vi "Shooter_Hood_Homing.vi"(0 "MotorConfig":T2={"CAN Address"=0, "Invert"=FALSE, "InvertSensor"=FALSE, "Unit Conversion Factor"=0.0, "Brake Mode"=enum."Override to Brake", "Reverse Limt Switch Mode"=enum."Disabled", "Forward Limt Swith Mode"=enum."Disabled", "PWM Channel"=enum."Invalid", "Motor Controller Type"=enum."Talon SRX", "Peak Current (A)"=0, "Continuous Current (A)"=0, "Peak Duration (ms)"=0, "Current Limit Enable"=FALSE}, 1 "Hood_Motor_DevRef":T7={"DeviceStatus"={"status"=FALSE, "code"=0, "source"=""}, "Type"=enum."PWM", "PWM"={"PWM Channel"=enum."Invalid", "DeadBand"={"Name"="", "maxPositivePwm"=0, "minPositivePwm"=0, "centerPwm"=0, "maxNegativePwm"=0, "minNegativePwm"=0, "angularRange"=0}}, "CAN"={"Device Number"=0, "SetOutput VI Ref"=variant(enum8{"Percent VBus", "Current", "Speed", "Position", "Voltage"} enum."Percent VBus"), "GetOutput VI Ref"=variant(refnum<k1> refnum), "Enable VI Ref"=variant(dbl 12.0), "Disable VI Ref"=variant(enum8{"Percent VBus", "Speed", "Position", "Slave", "Unchanged / Invalid", "Voltage Compensation", "Current", "Motion Profile"} enum."Percent VBus"), "Data"=variant}, "Invert"=FALSE, "DIO PWM"={"PWM \"Enable\" Channel"=enum."Invalid", "DIOChannel"=enum."Invalid", "PWM Rate"=0.0}}, 2 "Reset":bool, 3 "Homing Activated":bool, 4 "Controller_Command":dbl) -> (5 "Motor_Output":dbl, 6 "Homing_State":T1)   [LabVIEW 2019]
uses:
  <vilib>/Rock Robotics/WPI/MotorControl/WPI_MotorControlDeviceRef.ctl
  <vilib>/Rock Robotics/WPI/MotorControl/WPI_MotorControlType.ctl
  <vilib>/Rock Robotics/SystemInterfaces/DIO/FPGA_DIOPWMChannel.ctl
  <vilib>/Rock Robotics/WPI/PWM/WPI_PWMDeadband.ctl
  <vilib>/Rock Robotics/SystemInterfaces/DIO/FPGA_DIOChannel.ctl
  ArgosLib/Config/ConfigComponents/TypeDefs/Config_Motor.ctl
  <vilib>/Rock Robotics/WPI/ThirdParty/Phoenix-LabVIEW/Motor Controller/Controls/CTRE_Phoenix_MotorControl_NeutralMode.ctl
  <vilib>/Rock Robotics/WPI/ThirdParty/Phoenix-LabVIEW/Motor Controller/Controls/CTRE_Phoenix_MotorControl_LimitSwitchNormal.ctl
  ArgosLib/Config/ConfigComponents/TypeDefs/Config_MotorCtrlType.ctl
  TypeDefs/Hood_Homing_State.ctl
  ArgosLib/Signal Processing/TypeDefs/EdgeDetector_Type.ctl
  <vilib>/Rock Robotics/WPI/ThirdParty/Phoenix-LabVIEW/Motor Controller/Get/CTRE_Phoenix_MotorController_GetSupplyAndStatorCurrent_Enhanced.vi
  <vilib>/Rock Robotics/WPI/ThirdParty/Phoenix-LabVIEW/Motor Controller/Get/CTRE_Phoenix_MotorController_GetSelectedSensorData.vi
  ArgosLib/ArgosLib.lvlib
panel:
  in  "Command_Limit":dbl
  in  "Home_Position":dbl
  in  "Homing Speed":dbl=-0.1
  in  "Complete_Homing_Time (ms)":u32=250
  in  "Motor_Unresponsive_Time (ms)":u32=750
  in  "Stall_Current":dbl=0.5
  in  "Motor_Active_Current_Limit":dbl=0.05
  in  "Time_Out (ms)":u32=2500
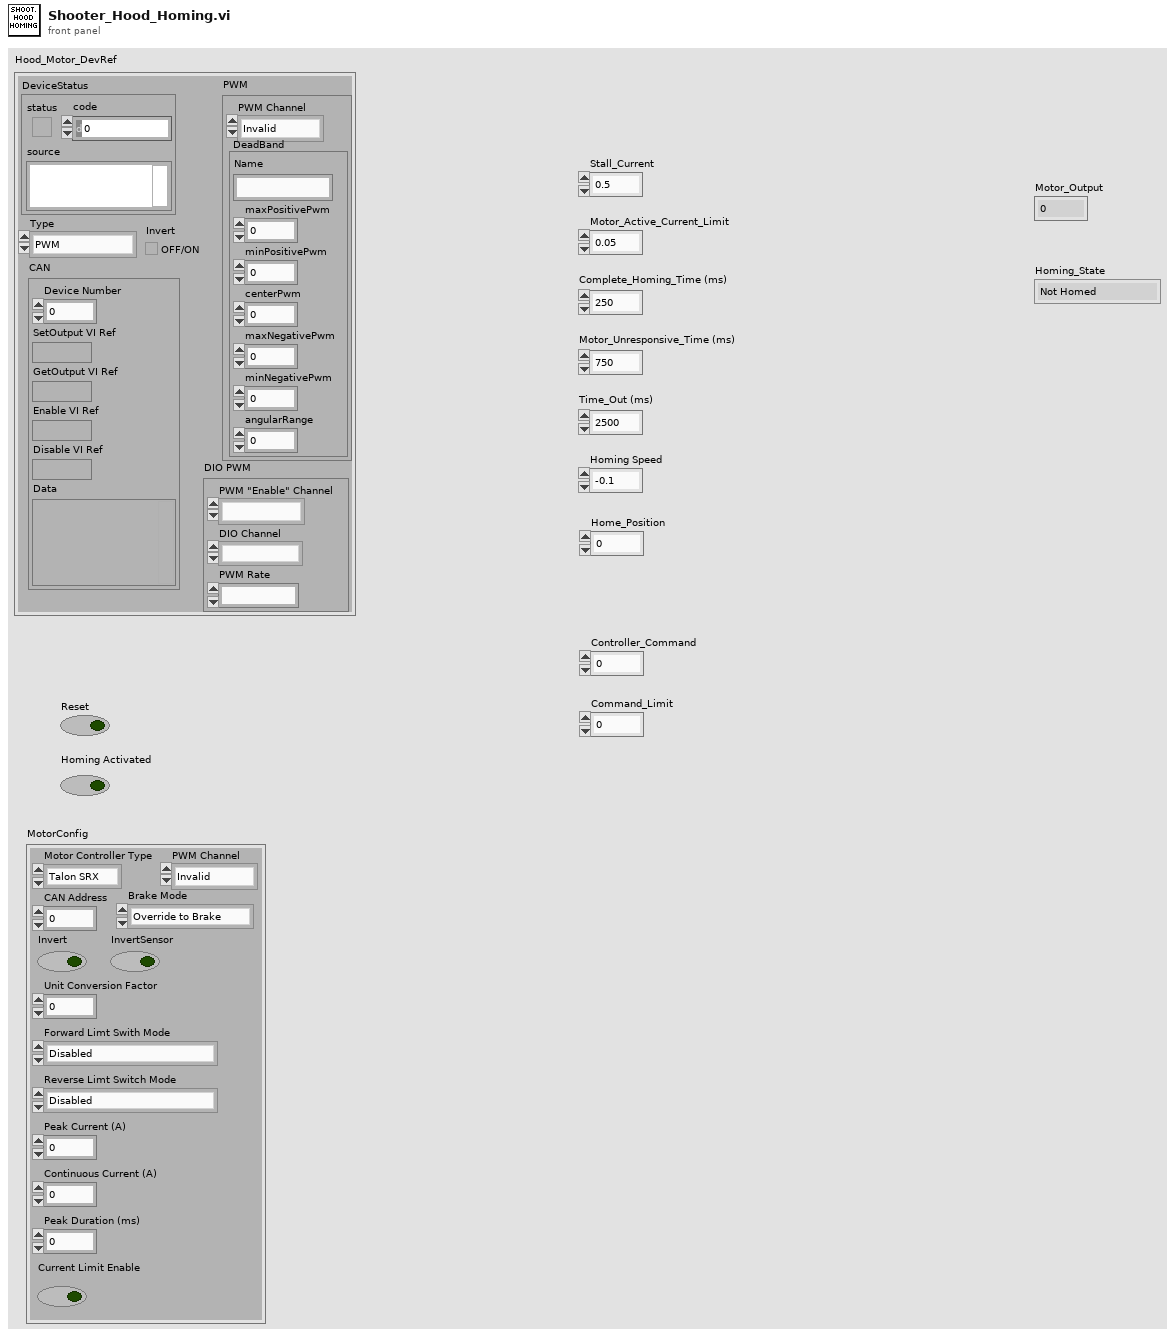
[diagram p1: front panel]
types:
  T1 = typedef "Hood_Homing_State.ctl" = enum16{"Not Homed", "Homing in Process", "Homing Failed", "Homing Completed"}
  T2 = typedef "ArgosLib.lvlib/Config_Motor.ctl" = cluster{"CAN Address":u8, "Invert":bool, "InvertSensor":bool, "Unit Conversion Factor":dbl, "Brake Mode":T3, "Reverse Limt Switch Mode":T4, "Forward Limt Swith Mode":T4, "PWM Channel":T5, "Motor Controller Type":T6, "Peak Current (A)":i32, "Continuous Current (A)":i32, "Peak Duration (ms)":i32, "Current Limit Enable":bool}
  T3 = typedef "CTRE_Phoenix_MotorControl_NeutralMode.ctl" = enum8{"EEPROMSetting", "Override to Coast", "Override to Brake"}
  T4 = typedef "CTRE_Phoenix_MotorControl_LimitSwitchNormal.ctl" = enum16{"Normally Open", "Normally Closed", "Disabled"}
  T5 = typedef "FPGA_DIOPWMChannel.ctl" = enum8{"PWM 0", "PWM 1", "PWM 2", "PWM 3", "PWM 4", "PWM 5", "PWM 6", "PWM 7", "PWM 8", "PWM 9", "PWM MXP 0", "PWM MXP 1", "PWM MXP 2", "PWM MXP 3", "PWM MXP 4", "PWM MXP 5", "PWM MXP 6", "PWM MXP 7", "PWM MXP 8", "PWM MXP 9", "Invalid"}
  T6 = typedef "ArgosLib.lvlib/Config_MotorCtrlType.ctl" = enum16{"Disabled", "Talon SRX", "Talon SR", "Venom", "Spark MAX"}
  T7 = typedef "WPI_MotorControlDeviceRef.ctl" = cluster{"DeviceStatus":errorcluster, "Type":T8, "PWM":cluster{"PWM Channel":T5, "DeadBand":T9}, "CAN":cluster{"Device Number":u8, "SetOutput VI Ref":variant, "GetOutput VI Ref":variant, "Enable VI Ref":variant, "Disable VI Ref":variant, "Data":variant}, "Invert":bool, "DIO PWM":cluster{"PWM \"Enable\" Channel":T5, "DIOChannel":T10, "PWM Rate":dbl}}
  T8 = typedef "WPI_MotorControlType.ctl" = enum16{"PWM", "CAN", "DIO PWM"}
  T9 = typedef "WPI_PWMDeadband.ctl" = cluster{"Name":string, "maxPositivePwm":i32, "minPositivePwm":i32, "centerPwm":i32, "maxNegativePwm":i32, "minNegativePwm":i32, "angularRange":u16}
  T10 = typedef "FPGA_DIOChannel.ctl" = enum8{"DIO 0", "DIO 1", "DIO 2", "DIO 3", "DIO 4", "DIO 5", "DIO 6", "DIO 7", "DIO 8", "DIO 9", "DIO MXP 0", "DIO MXP 1", "DIO MXP 2", "DIO MXP 3", "DIO MXP 4", "DIO MXP 5", "DIO MXP 6", "DIO MXP 7", "DIO MXP 8", "DIO MXP 9", "DIO MXP 10", "DIO MXP 11", "DIO MXP 12", "DIO MXP 13", "DIO MXP 14", "DIO MXP 15", "SPI Port CS1", "SPI Port CS2", "SPI Port CS3", "SPI Port MISO", "SPI Port MOSI", "Invalid"}
  T11 = typedef "ArgosLib.lvlib/EdgeDetector_Type.ctl" = enum16{"RisingEdge", "FallingEdge", "Both"}
  T12 = cluster{"Under Voltage":bool, "Forward Limit Switch":bool, "Reverse Limit Switch":bool, "Forward Soft Limit":bool, "Reverse Soft Limit":bool, "Hardware Failure":bool, "Reset During Enable":bool, "Sensor Overflow":bool, "Sensor Out of Phase":bool, "Hardware ESD Reset":bool, "Remote Loss of Signal":bool}
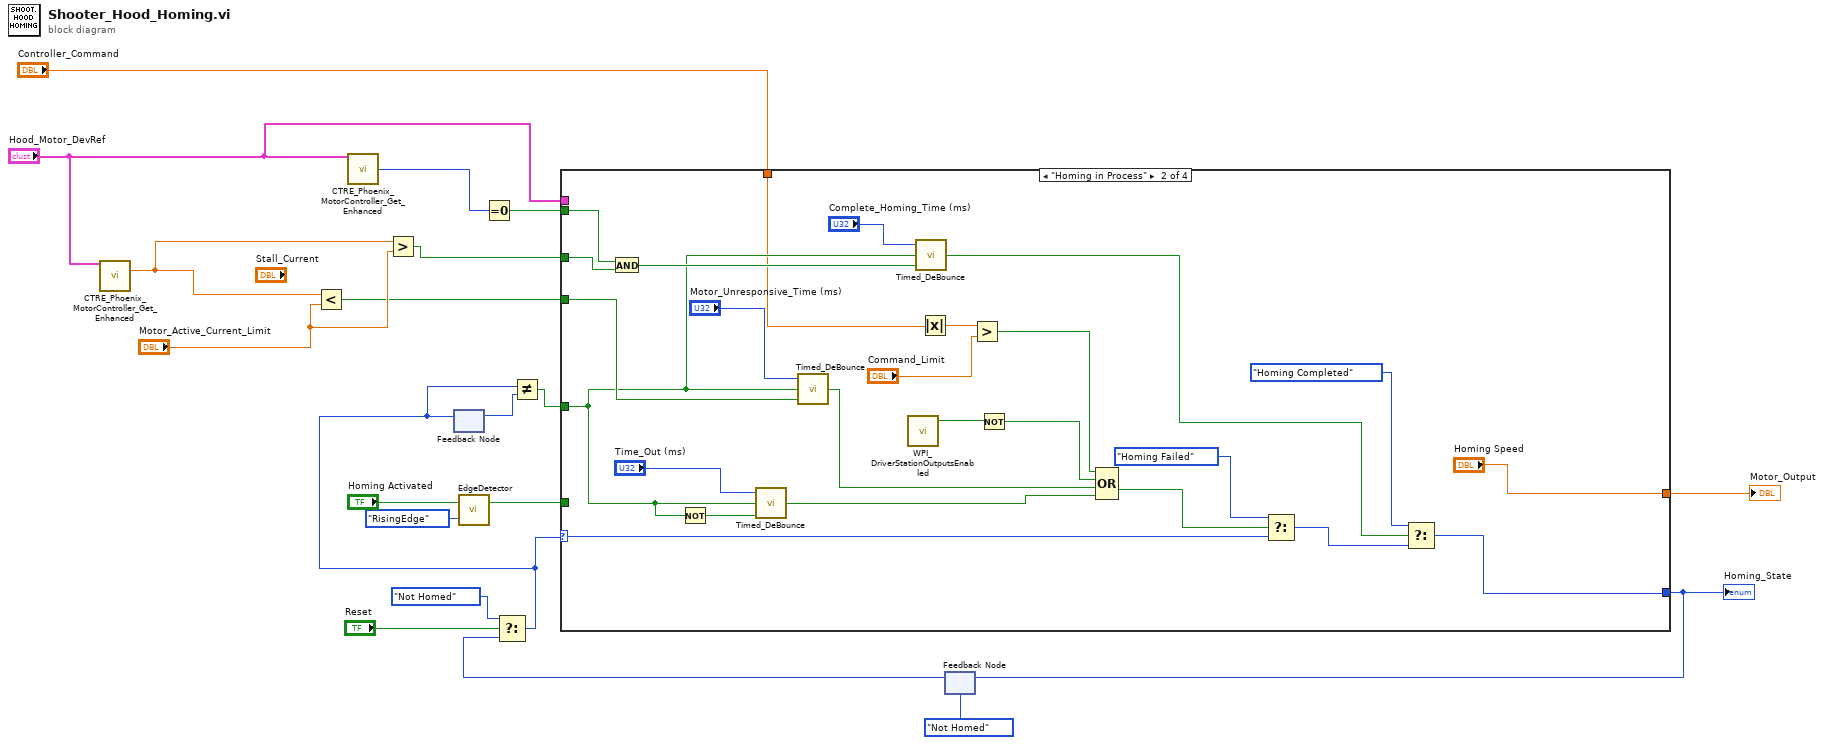
[diagram p0: block diagram]
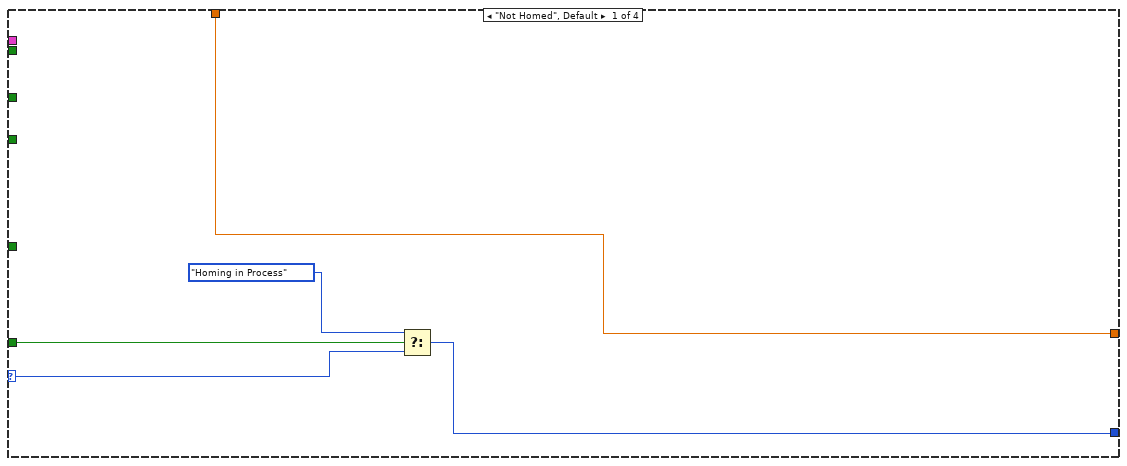
[diagram p2: hidden frame]
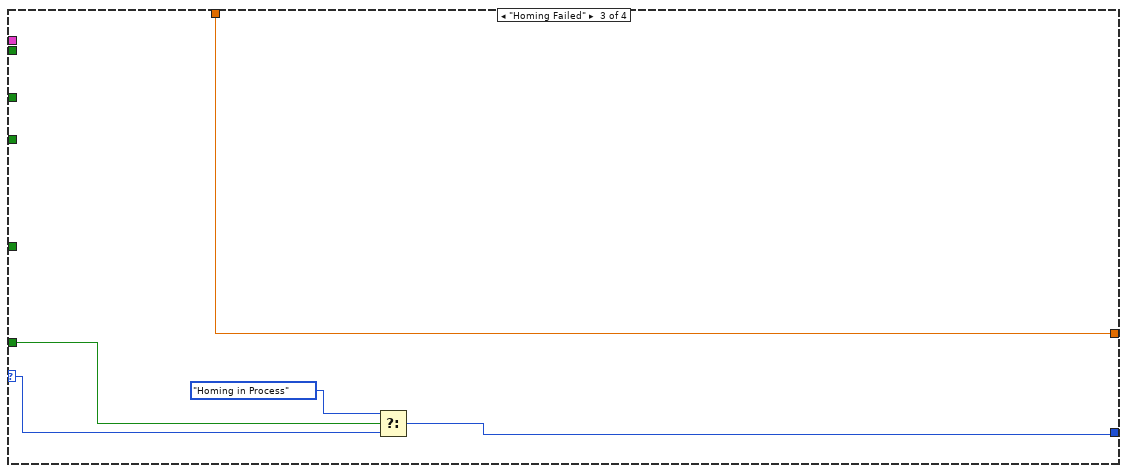
[diagram p3: hidden frame]
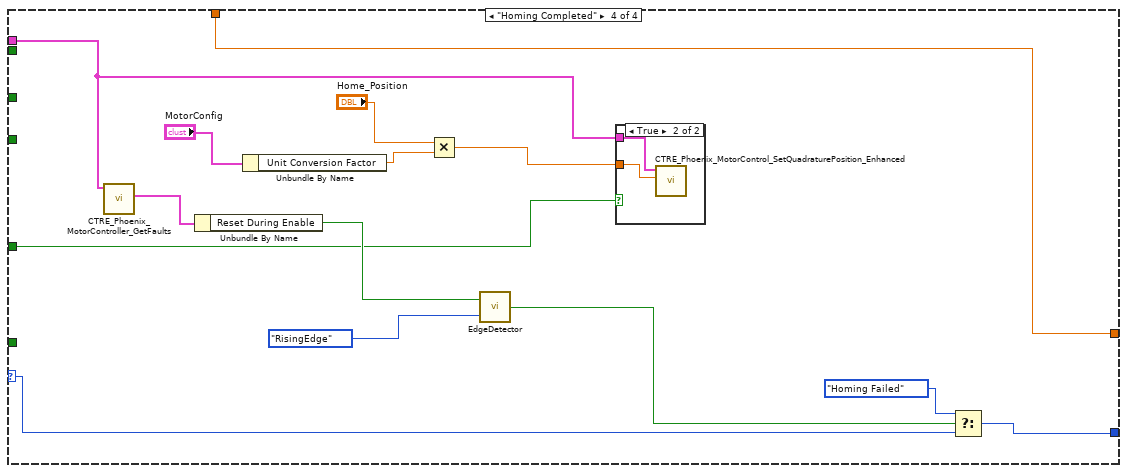
[diagram p4: hidden frame]
diagram:
  n1 = call-poly <vilib>:"CTRE_Phoenix_MotorController_Get_Enhanced.vi"("PhoenixMotorControlDevRef"="Hood_Motor_DevRef") -> ("Supply Current"=w11:dbl)  [unwired: 11 in, 3 out]
  n2 = Less?(x=w11, y="Motor_Active_Current_Limit") -> (x < y?=w2:bool)
  n3 = call-poly <vilib>:"CTRE_Phoenix_MotorController_Get_Enhanced.vi"("PhoenixMotorControlDevRef"="Hood_Motor_DevRef") -> ("Velocity (Raw Sensor Units per 100 ms)"=w10:i32)  [unwired: 11 in, 3 out]
  n4 = Greater?(x=w11, y="Motor_Active_Current_Limit") -> (0:w1:bool)
  n5 = feedback #1() -> (w14:T1)  [unwired: 1 in]
  n6 = call "EdgeDetector.vi"("DetectorType"=EdgeDetector_Type."RisingEdge", "Input"="Homing Activated") -> ("Edge"=w5:bool)
  n7 = Equal To 0?(x=w10) -> (x = 0?=w9:bool)
  n8 = feedback #2(Hood_Homing_State."Not Homed") -> (w18:T1)
  n9 = Select(t=Hood_Homing_State."Not Homed", s="Reset", f=w18) -> (s? t:f=w13:T1)
  n10 = feedback-in #1(w13) -> ()
  n11 = Not Equal?(x=w13, y=w14) -> (x != y?=w12:bool)
  n12 = case shown="\"Homing in Process\"" w13 {
    selector: w13 -> [w24 w48 w55 w59]
    tunnel: [w21 "Homing Speed" w51 w56] -> w7
    tunnel: w5 -> [w23 _ w52 _]
    tunnel: [w22 w50 w54 w69] -> w19
    tunnel: w12 -> [_ w31 _ w58]
    tunnel: w2 -> [_ w41 _ _]
    tunnel: w1 -> [_ w34 _ _]
    tunnel: w9 -> [_ w33 _ _]
    tunnel: "Hood_Motor_DevRef" -> [_ _ _ w57]
    tunnel: "Controller_Command" -> [w21 w26 w51 w56]
    frame "Not Homed", Default {
      n13 = Select(t=Hood_Homing_State."Homing in Process", s=w23, f=w24) -> (s? t:f=w22:T1)
    }
    frame "Homing in Process" {
      n14 = And(x=w33, y=w34) -> (x .and. y?=w32:bool)
      n15 = Not(x=w31) -> (.not. x?=w44:bool)
      n16 = call "Timed_DeBounce.vi"("Input"=w44, "Reset"=w31, "Hold Time(ms)"="Time_Out (ms)") -> ("Output"=w42:bool)
      n17 = call "Timed_DeBounce.vi"("Input"=w41, "Reset"=w31, "Hold Time(ms)"="Motor_Unresponsive_Time (ms)") -> ("Output"=w39:bool)
      n18 = call <vilib>:"WPI_DriverStationOutputsEnabled.vi"() -> ("OutputsEnabled?"=w37:bool)  [unwired: 10 in, 1 out]
      n19 = call "Timed_DeBounce.vi"("Input"=w32, "Reset"=w31, "Hold Time(ms)"="Complete_Homing_Time (ms)") -> ("Output"=w35:bool)
      n20 = Absolute Value(x=w26) -> (abs(x)=w29:dbl)
      n21 = Greater?(x=w29, y="Command_Limit") -> (0:w27:bool)
      n22 = Not(x=w37) -> (.not. x?=w38:bool)
      n23 = Compound Arithmetic op=OR(w27, w38, w39, w42) -> (w43:bool)
      n24 = Select(t=Hood_Homing_State."Homing Failed", s=w43, f=w48) -> (s? t:f=w47:T1)
      n25 = Select(t=Hood_Homing_State."Homing Completed", s=w35, f=w47) -> (s? t:f=w50:T1)
    }
    frame "Homing Failed" {
      n26 = Select(t=Hood_Homing_State."Homing in Process", s=w52, f=w55) -> (s? t:f=w54:T1)
    }
    frame "Homing Completed" {
      n27 = call <vilib>:"CTRE_Phoenix_MotorController_GetFaults.vi"("PhoenixMotorControlDevRef"=w57) -> ("Faults"=w66:T12)  [unwired: 8 in, 2 out]
      n28 = Unbundle By Name(w66) -> ("Reset During Enable"=w65:bool)
      n29 = Unbundle By Name("MotorConfig") -> ("Unit Conversion Factor"=w61:dbl)
      n30 = Multiply(x="Home_Position", y=w61) -> (x*y=w60:dbl)
      n31 = call "EdgeDetector.vi"("DetectorType"=EdgeDetector_Type."RisingEdge", "Input"=w65) -> ("Edge"=w67:bool)
      n32 = case shown="True" w58 {
        tunnel: w60 -> [_ w71]
        tunnel: w57 -> [_ w70]
        frame False {
        }
        frame True {
          n33 = call <vilib>:"CTRE_Phoenix_MotorControl_SetQuadraturePosition_Enhanced.vi"("New Position"=w71, "PhoenixMotorControlDevRef"=w70) -> ()  [unwired: 8 in, 2 out]
        }
      }
      n34 = Select(t=Hood_Homing_State."Homing Failed", s=w67, f=w59) -> (s? t:f=w69:T1)
    }
  }
  "Motor_Output" <- w7
  "Homing_State" <- w19
  n35 = feedback-in #2(w19) -> ()
